vi "Update Messages MetaData.vi"(7 "Messages MetaData":T1[](array[typedef]), 8 "error in (no error)":errorcluster, 11 "LVClassLibrary in":refnum<vi>) -> (0 "error out":errorcluster, 3 "LVClassLibrary out":refnum<vi>)   [LabVIEW 2019, in "gRPC Scripting Tools.lvlib"]
uses:
  gRPC Scripting Tools.lvlib
  TypeDefs/Message Metadata (Scripting).ctl
  TypeDefs/Message Element Metadata (Scripting).ctl
  TypeDefs/Message Element Type.ctl
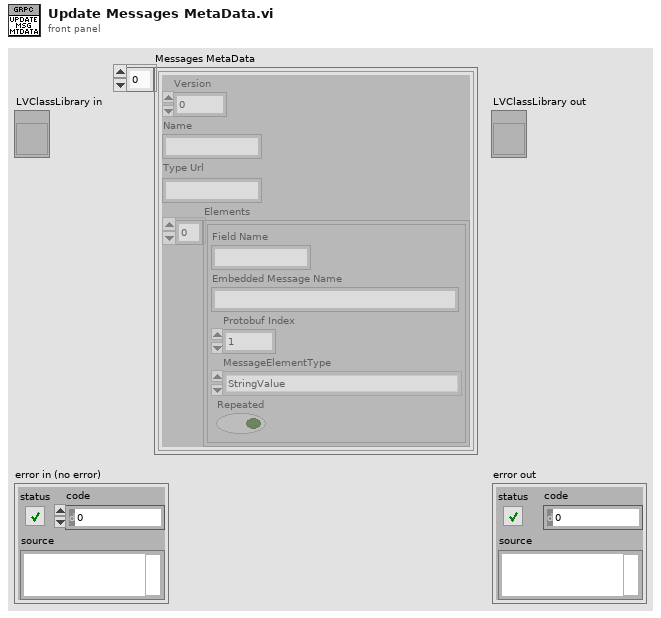
[diagram p1: front panel]
types:
  T1 = typedef "gRPC Scripting Tools.lvlib/Message Metadata (Scripting).ctl" = cluster{"Version":i32, "Name":string, "Type Url":string, "Elements":T2[]}
  T2 = typedef "gRPC Scripting Tools.lvlib/Message Element Metadata (Scripting).ctl" = cluster{"Field Name":string, "Embedded Message Name":string, "Protobuf Index":i32, "MessageElementType":T3, "Repeated":bool}
  T3 = typedef "gRPC Scripting Tools.lvlib/Message Element Type.ctl" = enum32{"Int32Value", "FloatValue", "DoubleValue", "BoolValue", "StringValue", "MessageValue", "Int64Value", "UInt32Value", "UInt64Value", "EnumValue", "Bytes", "Fixed64", "Fixed32", "SFixed64", "SFixed32", "SInt64", "SInt32"}
  T4 = cluster{"Version":i32, "Name":string, "Type Url":string, "Elements":cluster{"Embedded Message Name":string, "Protobuf Index":i32, "MessageElementType":enum32{"Int32Value", "FloatValue", "DoubleValue", "BoolValue", "StringValue", "MessageValue", "Int64Value", "UInt32Value", "UInt64Value", "EnumValue", "Bytes", "Fixed64", "Fixed32", "SFixed64", "SFixed32", "SInt64", "SInt32"}, "Repeated":bool}[]}
  T5 = cluster{"Embedded Message Name":string, "Protobuf Index":i32, "MessageElementType":enum32{"Int32Value", "FloatValue", "DoubleValue", "BoolValue", "StringValue", "MessageValue", "Int64Value", "UInt32Value", "UInt64Value", "EnumValue", "Bytes", "Fixed64", "Fixed32", "SFixed64", "SFixed32", "SInt64", "SInt32"}, "Repeated":bool}
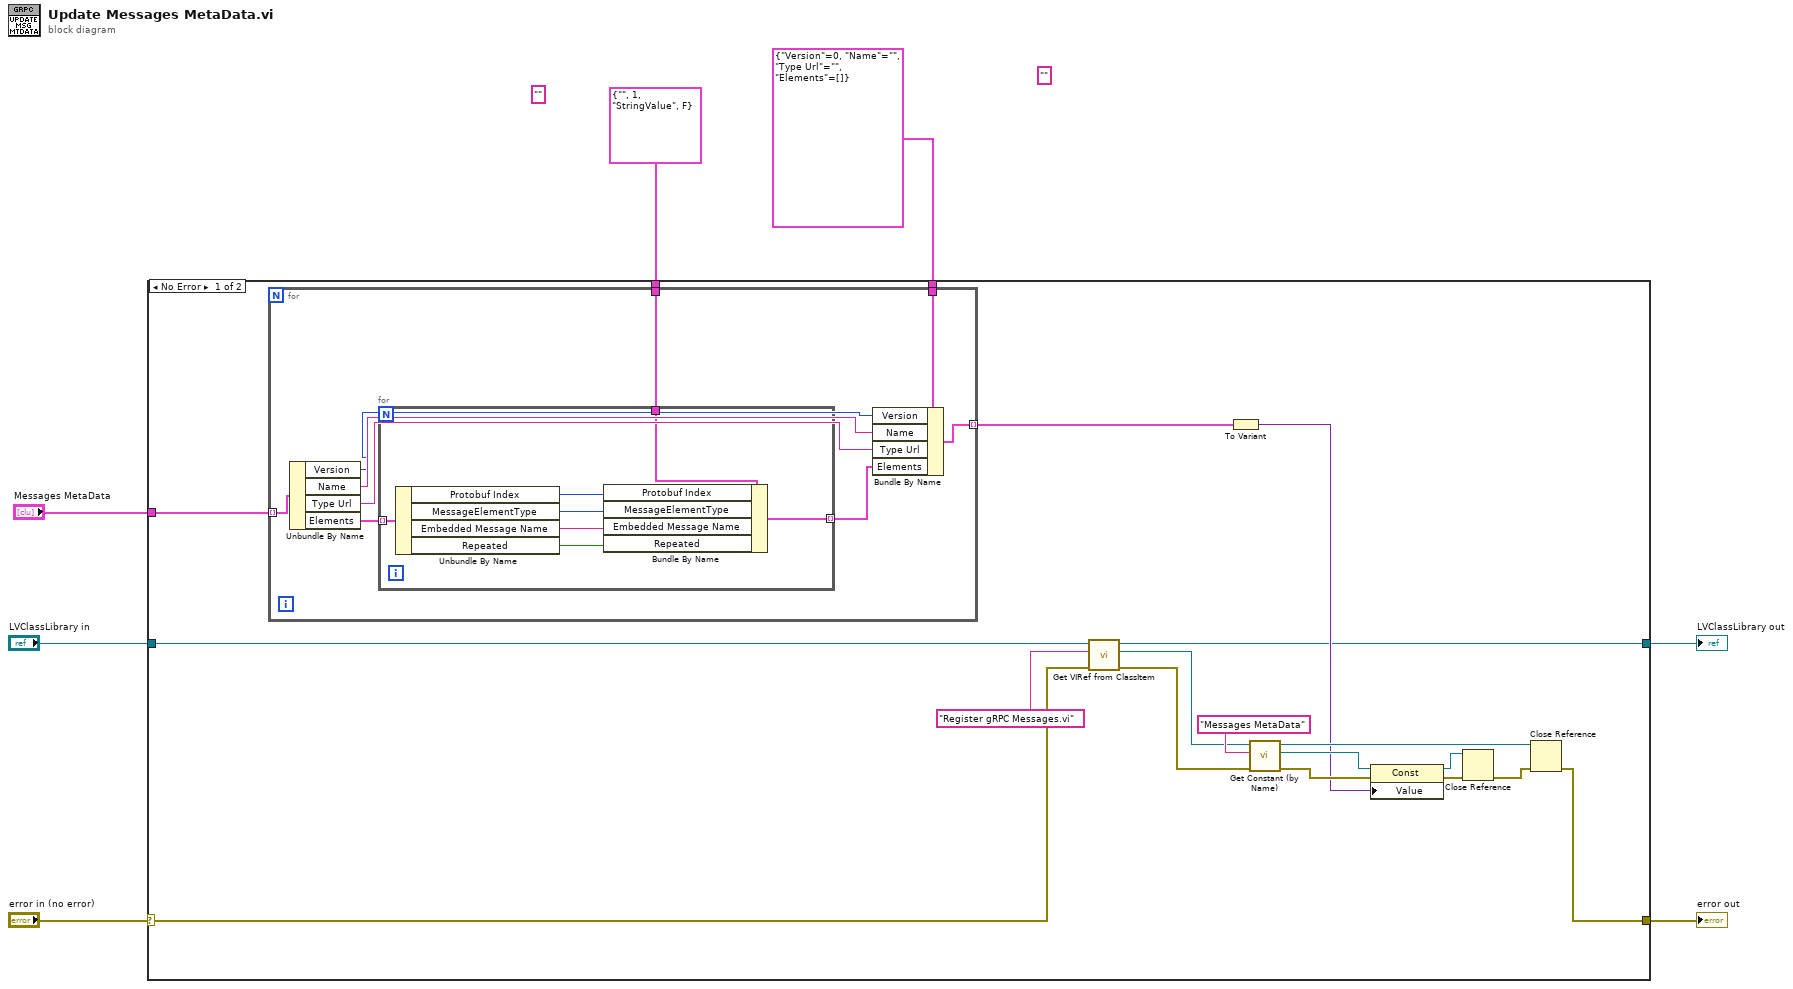
[diagram p0: block diagram]
diagram:
  (unwired) "" ("Field Name")
  (unwired) "" ("Field Name")
  n1 = case shown="No Error" "error in (no error)" {
    selector: "error in (no error)" -> [w12 w43]
    tunnel: [w26 w43] -> w7
    tunnel: [w15 w44] -> w6
    tunnel: "LVClassLibrary in" -> [w13 w44]
    tunnel: "Messages MetaData" -> [w11 _]
    tunnel: T5 {"Embedded Message Name"="", "Protobuf Index"=1, "MessageElementType"=enum."StringValue", "Repeated"=FALSE} ("Message Element Metadata") -> [w9 _]
    tunnel: T4 {"Version"=0, "Name"="", "Type Url"="", "Elements"=[]} ("Message Metadata") -> [w8 _]
    frame No Error {
      n2 = for {
        tunnel: w11 -> [w35] mode=indexing
        tunnel: [w33] -> w10 mode=indexing
        tunnel: w9 -> [w28]
        tunnel: w8 -> [w27]
        n3 = Unbundle By Name(w35) -> ("Version"=w29:i32, "Name"=w30:string, "Type Url"=w31:string, "Elements"=w34:T2[])
        n4 = for {
          tunnel: w34 -> [w42] mode=indexing
          tunnel: [w37] -> w32 mode=indexing
          tunnel: w28 -> [w36]
          n5 = Unbundle By Name(w42) -> ("Protobuf Index"=w41:i32, "MessageElementType"=w40:T3, "Embedded Message Name"=w39:string, "Repeated"=w38:bool)
          n6 = Bundle By Name(cluster=w36, "Protobuf Index"=w41, "MessageElementType"=w40, "Embedded Message Name"=w39, "Repeated"=w38) -> (w37:T5)
        }
        n7 = Bundle By Name(cluster=w27, "Version"=w29, "Name"=w30, "Type Url"=w31, "Elements"=w32) -> (w33:T4)
      }
      n8 = call "Get VIRef from ClassItem.vi"("error in (no error)"=w12, "Item Name"="Register gRPC Messages.vi", "LVClassLibrary in"=w13) -> ("error out"=w20:errorcluster, "VIref out"=w17:refnum<vi>, "LVClassLibrary out"=w15:refnum<vi>)  [unwired: 5 in, 1 out]
      n9 = To Variant(anything=w10) -> (Variant=w16:variant)
      n10 = call "Get Constant (by Name).vi"("error in (no error)"=w20, "Constant Label"="Messages MetaData", "Owner VI in"=w17) -> ("error out"=w21:errorcluster, "Const ref out"=w18:refnum<vi>, "Owner VI out"=w25:refnum<vi>)  [unwired: 5 in, 1 out]
      n11 = property class="Const"(reference=w18, error in=w21, "Value"=w16) -> (reference out=w23:refnum<vi>, error out=w22:errorcluster)
      n12 = Close Reference(reference=w23, error in (no error)=w22) -> (error out=w24:errorcluster)
      n13 = Close Reference(reference=w25, error in (no error)=w24) -> (error out=w26:errorcluster)
    }
    frame Error {
    }
  }
  "error out" <- w7
  "LVClassLibrary out" <- w6
